vi "Scale Variables.vi"(10 "Var 2":i16, 11 "Var 1":i16) -> (3 "Scaled output":i16)   [LabVIEW 2018, in "Control Box.lvlib" / "Control Box.lvclass"]
uses:
  Control Box.lvclass
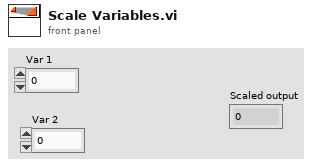
[diagram p1: front panel]
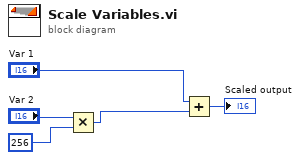
[diagram p0: block diagram]
diagram:
  n1 = Multiply(x="Var 2", y=i16 256) -> (x*y=w2:i16)
  n2 = Add(x="Var 1", y=w2) -> (x+y=→"Scaled output":i16)
